vi "California_housing.vi"(8 "error in (no error)":errorcluster caption="entrée d'erreur (pas d'erreur)", 11 "fetch_california_housing":T2={"download_if_missing"=TRUE, "Returns"="Data"}) -> (0 "error out":errorcluster, 3 "Data":T1)   [LabVIEW 2020]
doc: "This dataset was derived from the 1990 U.S. census, using one row per census block group. A block group is the smallest geographical unit for which the U.S. Census Bureau publishes sample data (a block group typically has a population of 600 to 3,000 people).\n\nParameters : \n\n- download_if_missingoptional, default=True\n If False, raise a IOError if the data is not locally available instead of trying to download the data from the source site.\n\nReturns : \n\n- data : ndarray, shape (20640, 8)\nEach row corresponding to the 8 feature values in order. If as_frame is True, data is a pandas object.\n\n- target : numpy array of shape (20640,)\nEach value corresponds to the average house value in units of 100,000. If as_frame is True, target is a pandas object.\n\n\n\nData Set Characteristics :\n\nNumber of Instances : 20640\n\nNumber of Attributes : 8 numeric, predictive attributes and the target\n\nAttribute Information : \n - MedInc median income in block\n - HouseAge median house age in block\n - AveRooms average number of rooms\n - AveBedrms average number of bedrooms\n - Population block population\n - AveOccup average house occupancy\n - Latitude house block latitude\n - Longitude house block longitude\n\nMissing Attribute Values : None\n\n\nThe target variable is the median house value for California districts."
uses:
  California_housing.lvclass
panel:
  out "California_housing.lvclass":refnum<class "California_housing.lvclass">
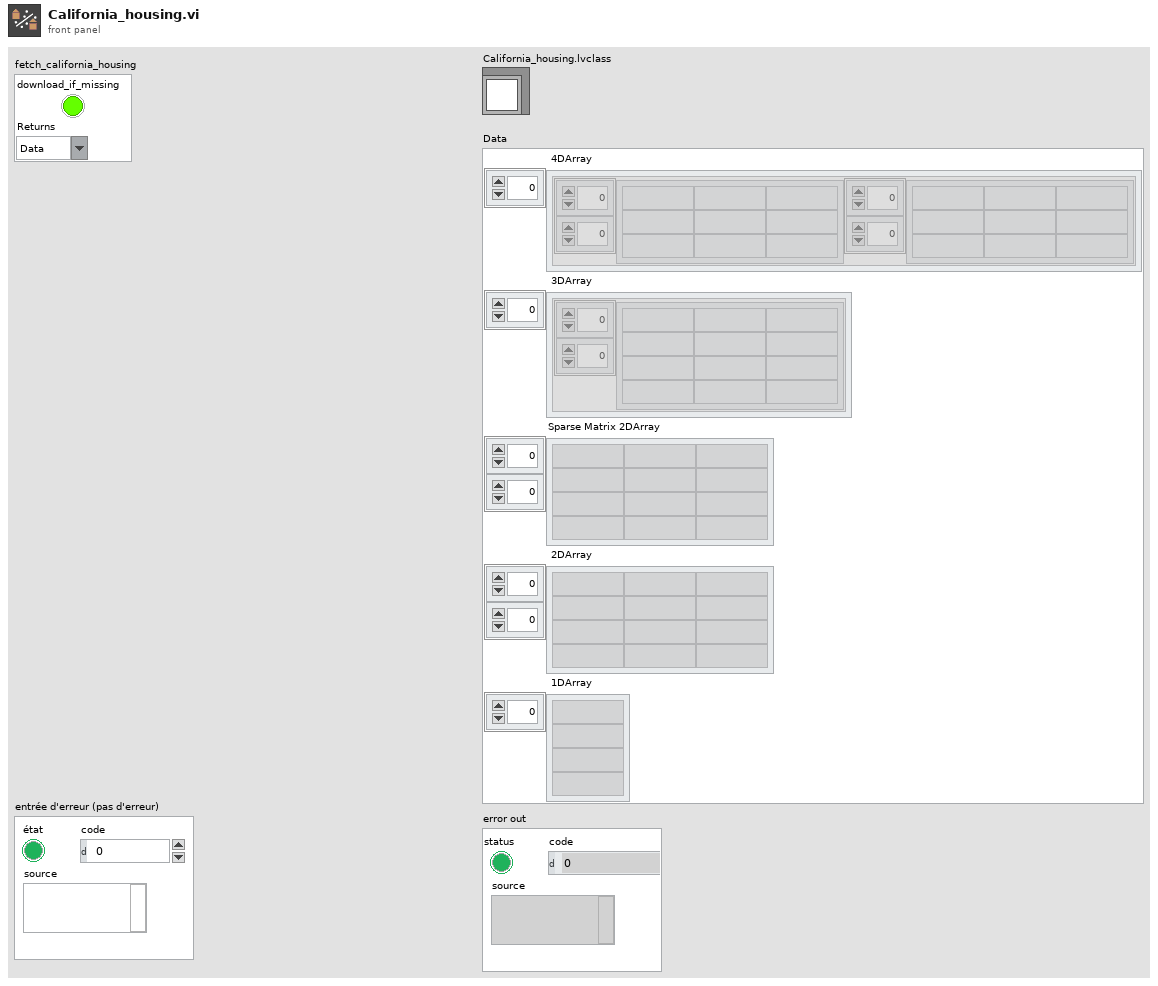
[diagram p1: front panel]
types:
  T1 = cluster{" 4DArray":cluster{"1":string[][], "2":string[][]}[], " 3DArray":cluster{"Tableau":string[][]}[], "Sparse Matrix 2DArray":string[][], " 2DArray":string[][], " 1DArray":string[]}
  T2 = cluster{"download_if_missing":bool, "Returns":string}
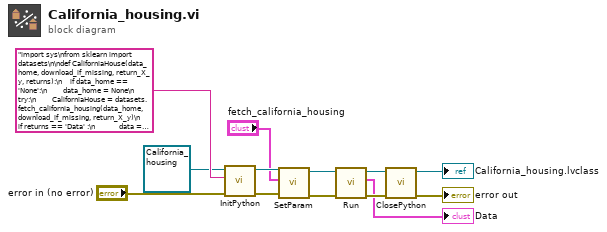
[diagram p0: block diagram]
diagram:
  n1 = call-dynamic "InitPython.vi"("error in (no error)"="error in (no error)", "Python Instruction"="import sys\nfrom sklearn import datasets\n\ndef CaliforniaHouse(data_home, download_if_missing, return_X_y, returns):\n    if data_home == 'None':\n        data_home = None\n    try:\n        CaliforniaHouse = datasets.fetch_california_housing(data_home, download_if_missing, return_X_y)\n        if returns == 'Data' :\n            data = CaliforniaHouse['data'].tolist()\n            return str(data)\n        else :\n            data = CaliforniaHouse['target'].tolist()\n            return str(data)\n    except:\n        erreur = sys.exc_info()\n        typerr = u\"%s\" % (erreur[0])\n        typerr = typerr[typerr.find(\"'\")+1:typerr.rfind(\"'\")]\n        msgerr = u\"%s\" % (erreur[1])\n        message = str('/!\\\\ {0} : {1}'. format(typerr,msgerr))\n        return message", "Scikit-learn en entrée"=refnum<class "California_housing.lvclass"> refnum ("California_housing.lvclass")) -> ("error out"=w8:errorcluster, "Scikit-learn en sortie"=w11:refnum<class "California_housing.lvclass">)  [unwired: 7 in]
  n2 = call-dynamic "SetParam.vi"("error in (no error)"=w8, "fetch_california_housing"="fetch_california_housing", "California_housing.lvclass"=w11) -> ("error out"=w6:errorcluster, "California_housing.lvclass"=w7:refnum<class "California_housing.lvclass">)  [unwired: 7 in]
  n3 = call-dynamic "Run.vi"("error in (no error)"=w6, "California_housing.lvclass"=w7) -> ("error out"=w4:errorcluster, "Data"=→"Data":T1, "California_housing.lvclass"=w5:refnum<class "California_housing.lvclass">)  [unwired: 7 in]
  n4 = call-dynamic "ClosePython.vi"("error in (no error)"=w4, "Scikit-learn en entrée"=w5) -> ("error out"=→"error out":errorcluster, "Scikit-learn en sortie"=→"California_housing.lvclass":refnum<class "California_housing.lvclass">)  [unwired: 8 in]
